vi "Set Build Spec Absolute Paths.vi"(8 "error in":errorcluster, 9 "Destination[i] Paths (Absolute)":path[](array[path]), 10 "LocalDestDir (Absolute)":path, 11 "Build Spec":refnum<vi>) -> (0 "error out":errorcluster, 3 "Build Spec (dup)":refnum<vi>)   [LabVIEW 2021]
doc: "Set the absolute destination paths of a build specification.\n\nMade by raphschru for the NI forum."
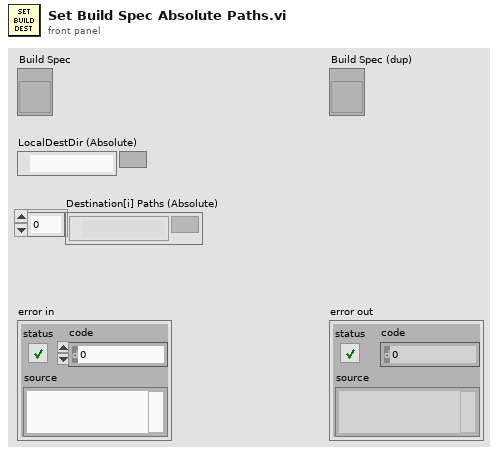
[diagram p1: front panel]
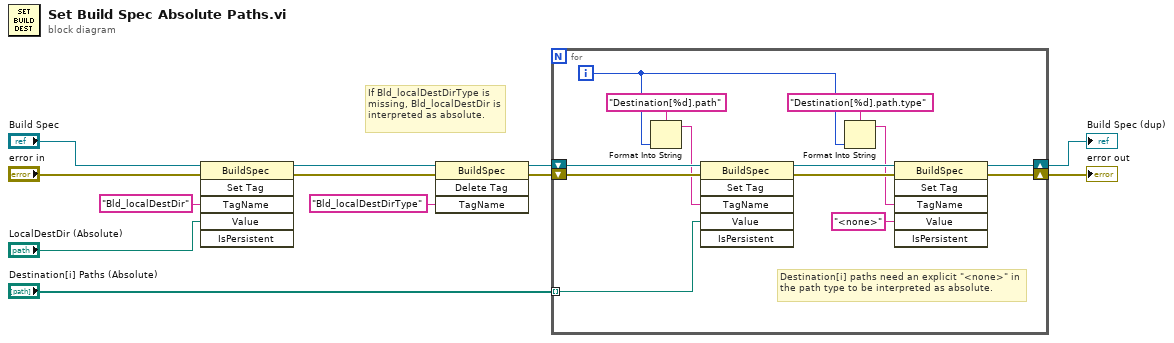
[diagram p0: block diagram]
diagram:
  # "If Bld_localDestDirType is missing, Bld_localDestDir is interpreted as absolute."
  n1 = invoke class="BuildSpec" method="Set Tag"(reference="Build Spec", error in="error in", "TagName"="Bld_localDestDir" ("Tag Name"), "Value"="LocalDestDir (Absolute)") -> (reference out=w10:refnum<vi>, error out=w3:errorcluster)  [unwired: 2 in, 4 out]
  n2 = invoke class="BuildSpec" method="Delete Tag"(reference=w10, error in=w3, "TagName"="Bld_localDestDirType" ("Tag Name")) -> (reference out=w9:refnum<vi>, error out=w2:errorcluster)  [unwired: 1 in, 2 out]
  n3 = for {
    tunnel: "Destination[i] Paths (Absolute)" -> [w20] mode=indexing
    shift-right: [w23] -> w4
    shift-left: w9 -> [w25]
    shift-right: [w17] -> w1
    shift-left: w2 -> [w19]
    i -> [w13]
    # "Destination[i] paths need an explicit \"<none>\" in the path type to be interpreted as absolute."
    n4 = Format Into String(format string="Destination[%d].path", w13) -> (resulting string=w14:string)  [unwired: 2 in, 1 out]
    n5 = invoke class="BuildSpec" method="Set Tag"(reference=w25, error in=w19, "TagName"=w14, "Value"=w20) -> (reference out=w24:refnum<vi>, error out=w18:errorcluster)  [unwired: 2 in, 4 out]
    n6 = Format Into String(format string="Destination[%d].path.type", w13) -> (resulting string=w15:string)  [unwired: 2 in, 1 out]
    n7 = invoke class="BuildSpec" method="Set Tag"(reference=w24, error in=w18, "TagName"=w15, "Value"="<none>") -> (reference out=w23:refnum<vi>, error out=w17:errorcluster)  [unwired: 2 in, 4 out]
  }
  "Build Spec (dup)" <- w4
  "error out" <- w1
